vi "test 12- workerModeCallsChainMode.vi"(8 "error in (no error)":errorcluster, 11 "TestCase in":refnum<class "testcase-SyncMessage.lvclass">) -> (0 "error out":errorcluster, 3 "TestCase out":refnum<class "testcase-SyncMessage.lvclass">)   [LabVIEW 2017, in "testcase-SyncMessage.lvclass"]
uses:
  testcase-SyncMessage.lvclass
  <vilib>/addons/_JKI Toolkits/VI Tester/TestCase.llb/TestCase.lvclass
  src/user.lib/_NEVSTOP/Communicable State Machine(CSM)/Communicable State Machine.lvlib
  C:/Program Files (x86)/National Instruments/LabVIEW 2017/vi.lib/addons/_JKI Toolkits/VI Tester/TestCase.llb/TestCase.lvclass
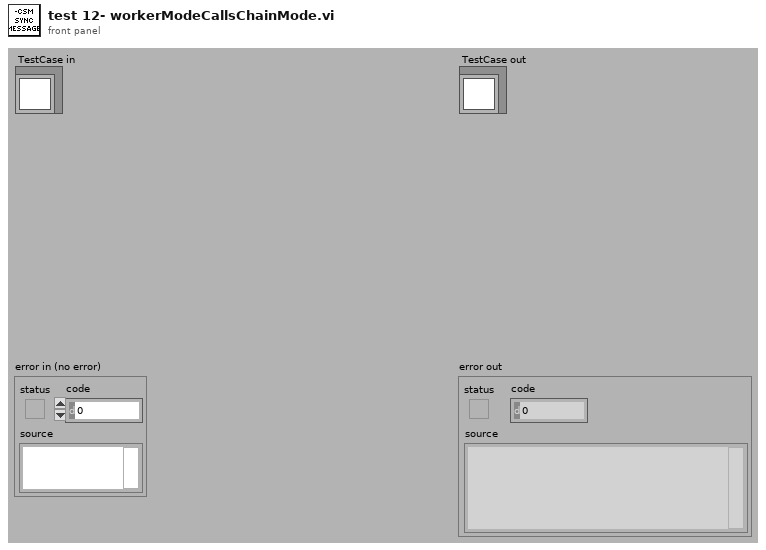
[diagram p1: front panel]
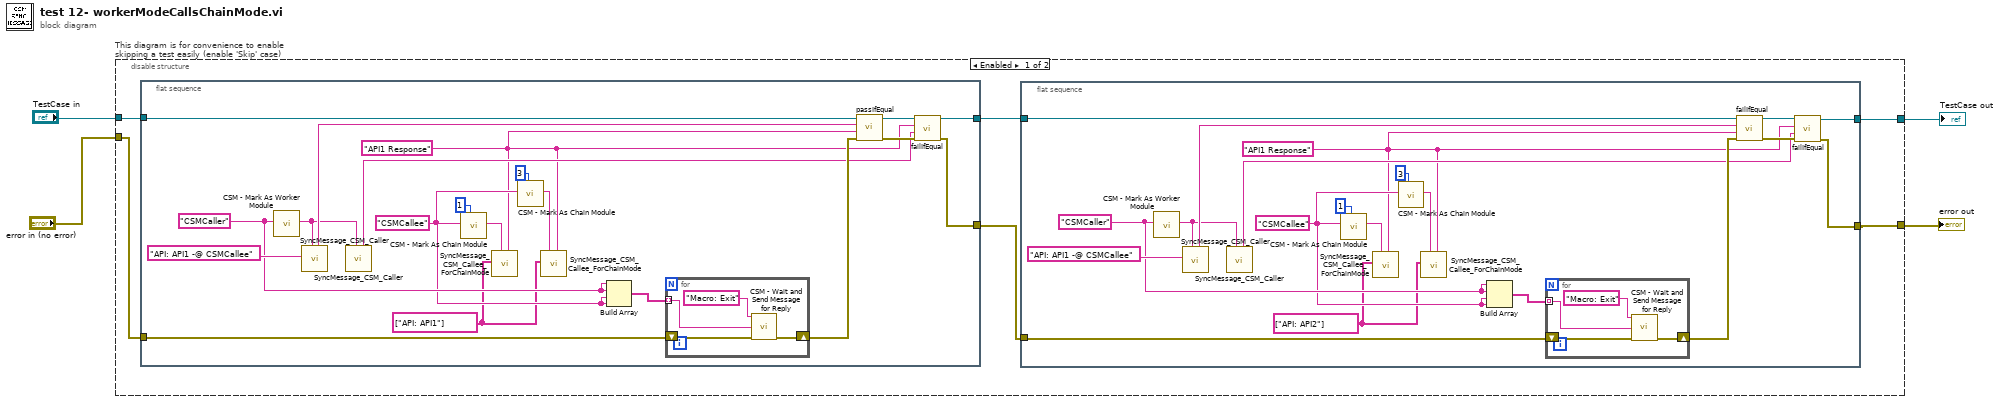
[diagram p0: block diagram]
diagram:
  n1 = disable-structure "This diagram is for convenience to enable skipping a test easily (enable 'Skip' case)" shown="Enabled" {
    disable-tunnel: "TestCase in" -> [w10 w62]
    disable-tunnel: [w7 w60] -> w2
    disable-tunnel: [w5 w61] -> w1
    disable-tunnel: "error in (no error)" -> [w9 w59]
    frame Enabled {
      n2 = flat-sequence {
        tunnel: w10 -> [w54]
        tunnel: w9 -> [w49]
        tunnel: [w45] -> w8
        tunnel: [w43] -> w6
        frame #0 {
          w35 = string[] ["API: API1"] ("Allowed Messages (Empty for All)")
          w39 = "CSMCallee" ("CSMCallee")
          w47 = "CSMCaller" ("CSMCaller")
          w36 = "API1 Response" ("API response in")
          n3 = call "CSM - Mark As Worker Module.vi"("CSM Name"=w47) -> ("CSM Name (Marked As Worker)"=w48:string)  [unwired: 9 in]
          n4 = call "SyncMessage_CSM_Caller.vi"("Name (\"\" to Use UUID)"=w48, "Intermodule Message in"="API: API1 -@ CSMCallee") -> ("API received Response out"=w52:string)  [unwired: 9 in]
          n5 = call "SyncMessage_CSM_Caller.vi"("Name (\"\" to Use UUID)"=w48) -> ("API received Response out"=w42:string)  [unwired: 10 in]
          n6 = call "CSM - Mark As Chain Module.vi"("Order"=1, "CSM Name"=w39) -> ("CSM Name (Marked As Chain)"=w38:string)  [unwired: 8 in]
          n7 = call "SyncMessage_CSM_Callee_ForChainMode.vi"("API response in"=w36, "Name (\"\" to Use UUID)"=w38, "Allowed Messages (Empty for All)"=w35) -> ()  [unwired: 9 in]
          n8 = call "CSM - Mark As Chain Module.vi"("Order"=3, "CSM Name"=w39) -> ("CSM Name (Marked As Chain)"=w37:string)  [unwired: 8 in]
          n9 = call "SyncMessage_CSM_Callee_ForChainMode.vi"("API response in"=w36, "Name (\"\" to Use UUID)"=w37, "Allowed Messages (Empty for All)"=w35) -> ()  [unwired: 9 in]
          n10 = Build Array(w47, w47, w39, w39) -> (w51:string[])
          n11 = for {
            shift-right: [w56] -> w50
            shift-left: w49 -> [w57]
            tunnel: w51 -> [w55] mode=indexing
            n12 = call "CSM - Wait and Send Message for Reply.vi"("State"="Macro: Exit", "Target Module"=w55, "Error In (No Error)"=w57) -> ("error out"=w56:errorcluster)  [unwired: 10 in, 2 out]
          }
          n13 = call-dynamic "passIfEqual.vi"("error in (no error)"=w50, "y"=w36, "x"=w52, "TestCase in"=w54) -> ("error out"=w44:errorcluster, "TestCase out"=w46:refnum<class "testcase-SyncMessage.lvclass">)  [unwired: 6 in]
          n14 = call-dynamic "failIfEqual.vi"("error in (no error)"=w44, "y"=w42, "x"=w36, "TestCase in"=w46) -> ("error out"=w43:errorcluster, "TestCase out"=w45:refnum<class "testcase-SyncMessage.lvclass">)  [unwired: 6 in]
        }
      }
      n15 = flat-sequence {
        tunnel: w8 -> [w30]
        tunnel: w6 -> [w25]
        tunnel: [w21] -> w7
        tunnel: [w19] -> w5
        frame #0 {
          w11 = string[] ["API: API2"] ("Allowed Messages (Empty for All)")
          w15 = "CSMCallee" ("CSMCallee")
          w23 = "CSMCaller" ("CSMCaller")
          w12 = "API1 Response" ("API response in")
          n16 = call "CSM - Mark As Worker Module.vi"("CSM Name"=w23) -> ("CSM Name (Marked As Worker)"=w24:string)  [unwired: 9 in]
          n17 = call "SyncMessage_CSM_Caller.vi"("Name (\"\" to Use UUID)"=w24, "Intermodule Message in"="API: API1 -@ CSMCallee") -> ("API received Response out"=w28:string)  [unwired: 9 in]
          n18 = call "SyncMessage_CSM_Caller.vi"("Name (\"\" to Use UUID)"=w24) -> ("API received Response out"=w18:string)  [unwired: 10 in]
          n19 = call "CSM - Mark As Chain Module.vi"("Order"=1, "CSM Name"=w15) -> ("CSM Name (Marked As Chain)"=w14:string)  [unwired: 8 in]
          n20 = call "SyncMessage_CSM_Callee_ForChainMode.vi"("API response in"=w12, "Name (\"\" to Use UUID)"=w14, "Allowed Messages (Empty for All)"=w11) -> ()  [unwired: 9 in]
          n21 = call "CSM - Mark As Chain Module.vi"("Order"=3, "CSM Name"=w15) -> ("CSM Name (Marked As Chain)"=w13:string)  [unwired: 8 in]
          n22 = call "SyncMessage_CSM_Callee_ForChainMode.vi"("API response in"=w12, "Name (\"\" to Use UUID)"=w13, "Allowed Messages (Empty for All)"=w11) -> ()  [unwired: 9 in]
          n23 = Build Array(w23, w23, w15, w15) -> (w27:string[])
          n24 = for {
            shift-right: [w32] -> w26
            shift-left: w25 -> [w33]
            tunnel: w27 -> [w31] mode=indexing
            n25 = call "CSM - Wait and Send Message for Reply.vi"("State"="Macro: Exit", "Target Module"=w31, "Error In (No Error)"=w33) -> ("error out"=w32:errorcluster)  [unwired: 10 in, 2 out]
          }
          n26 = call-dynamic "failIfEqual.vi"("error in (no error)"=w26, "y"=w12, "x"=w28, "TestCase in"=w30) -> ("error out"=w20:errorcluster, "TestCase out"=w22:refnum<class "testcase-SyncMessage.lvclass">)  [unwired: 6 in]
          n27 = call-dynamic "failIfEqual.vi"("error in (no error)"=w20, "y"=w18, "x"=w12, "TestCase in"=w22) -> ("error out"=w19:errorcluster, "TestCase out"=w21:refnum<class "testcase-SyncMessage.lvclass">)  [unwired: 6 in]
        }
      }
    }
    frame Disabled {
      # "skip test result while test is under development"
      n28 = call <vilib>:"skip.vi"("error in (no error)"=w59, "TestCase in"=w62) -> ("error out"=w61:errorcluster, "TestCase out"=w60:refnum<class "testcase-SyncMessage.lvclass">)  [unwired: 8 in]
    }
  }
  "error out" <- w1
  "TestCase out" <- w2
